vi "String Ends With.vi"(7 "ignore case? (f: case sensitive)":bool, 9 "ending":string, 11 "string":string) -> (2 "ends with?":bool)   [LabVIEW 2020, in "JKI JSON Object Serialization.lvlib" / "OOP_Utility.lvlib"]
uses:
  OOP_Utility.lvlib
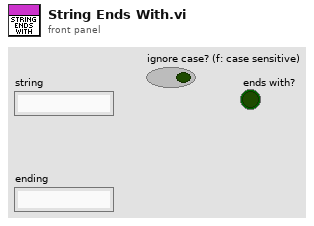
[diagram p1: front panel]
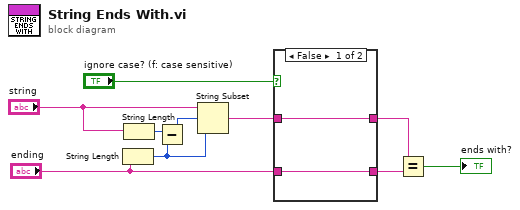
[diagram p0: block diagram]
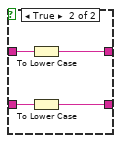
[diagram p2: hidden frame]
diagram:
  n1 = String Length(string="ending") -> (length=w4:i32)
  n2 = String Length(string="string") -> (length=w2:i32)
  n3 = Subtract(x=w2, y=w4) -> (x-y=w3:i32)
  n4 = String Subset(string="string", offset (0)=w3, length (rest)=w4) -> (substring=w5:string)
  n5 = case shown="False" "ignore case? (f: case sensitive)" {
    tunnel: [w11 w16] -> w10
    tunnel: [w12 w15] -> w8
    tunnel: "ending" -> [w11 w14]
    tunnel: w5 -> [w12 w13]
    frame False {
    }
    frame True {
      n6 = To Lower Case(string=w13) -> (all lower case string=w15:string)
      n7 = To Lower Case(string=w14) -> (all lower case string=w16:string)
    }
  }
  n8 = Equal?(x=w8, y=w10) -> (x = y?=→"ends with?":bool)
